vi "Set Param.vi"(4 "error in (no error)":errorcluster, 6 "param":dbl, 7 "paramID":i32) -> (0 "error out":errorcluster, 3 "function return":i32)   [LabVIEW 2020, in "MPH16.lvlib"]
doc: "long SetParam(const long paramID, const double param);"
uses:
  MPH16.lvlib
  ThorPinholeStepper.dll
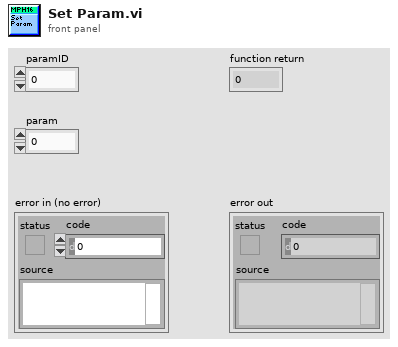
[diagram p1: front panel]
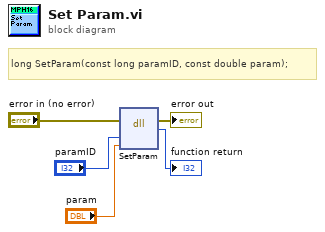
[diagram p0: block diagram]
diagram:
  # "long SetParam(const long paramID, const double param);"
  n1 = dll-call lib="D:/software/TweezerTron/ThorPinholeStepper.*" fn="SetParam"(error in="error in (no error)", "paramID"="paramID", "param"="param") -> (error out=→"error out":errorcluster, →"function return":i32)  [unwired: 4 in, 1 out]
